vi "Load_from_Project.vi"(8 "error in (no error)":errorcluster, 9 "index":string, 10 "buildObject":T1, 11 "Class in":refnum<class "IB_DistPart.lvclass">) -> (0 "error out":errorcluster, 3 "Class out":refnum<class "IB_DistPart.lvclass">)   [LabVIEW 2020, in "IB_DistPart.lvclass"]
uses:
  <vilib>/AppBuilder/IB_Classes/DistPart/IB_DistPart.lvclass
  <vilib>/AppBuilder/IB_Classes/DistPart/IB_DistPart.lvclass/IB_DistPart.ctl
  <vilib>/AppBuilder/IB_RW_Project/IB_RW_Project_PropBag_Action.ctl
  <vilib>/AppBuilder/IB_Classes/SoftDependency/IB_SoftDependency.lvclass
  <resource>/Framework/Providers/API/ItemRef.ctl
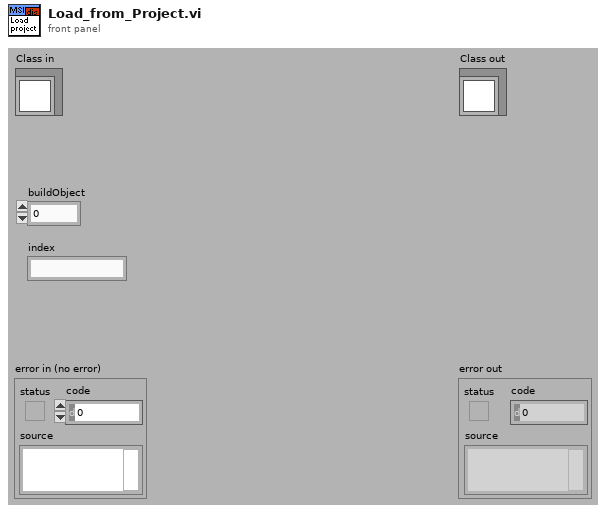
[diagram p1: front panel]
types:
  T1 = typedef "ItemRef.ctl" = u64
  T2 = typedef "IB_RW_Project_PropBag_Action.ctl" = enum16{"read", "write", "clear", "readPrevious", "writePrevious", "clearPrevious"}
  T3 = typedef "IB_RW_Project_DistPart_Data.ctl" = cluster{"ProductId":string, "FlavorId":string, "ProdName":string, "UpgradeCode":string}
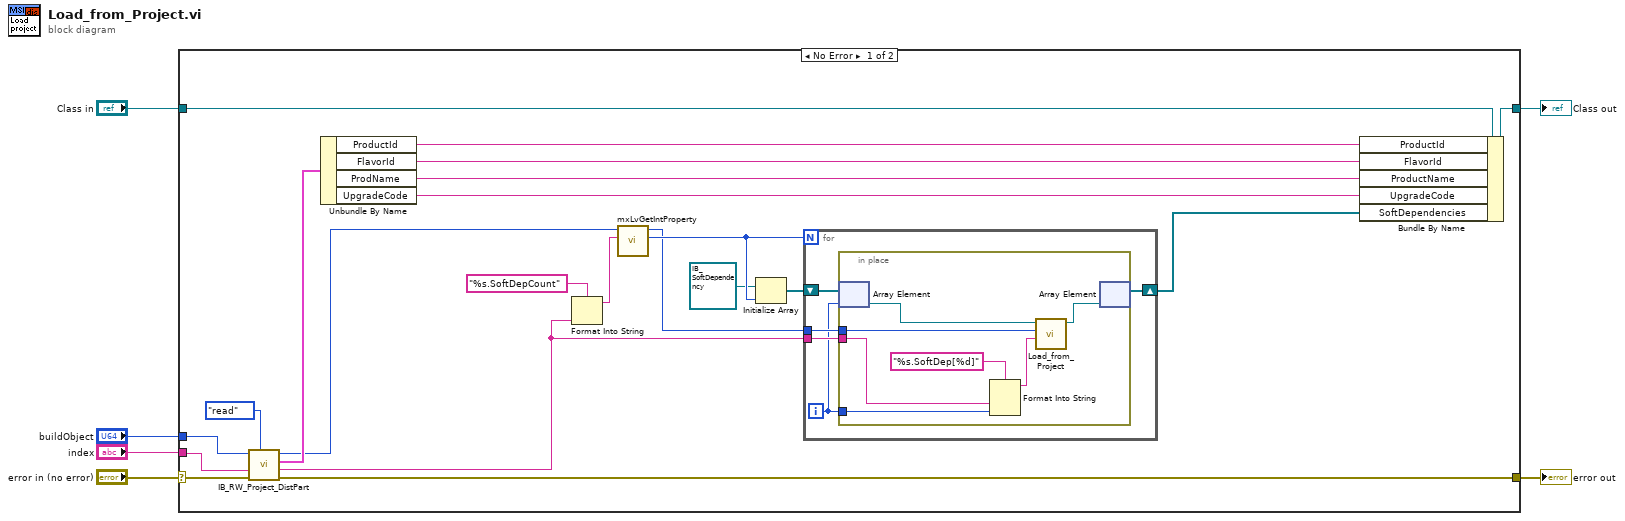
[diagram p0: block diagram]
diagram:
  n1 = case shown="No Error" "error in (no error)" {
    selector: "error in (no error)" -> [w17 w41]
    tunnel: [w16 w41] -> w5
    tunnel: [w23 w40] -> w3
    tunnel: "Class in" -> [w24 w40]
    tunnel: "buildObject" -> [w27 _]
    tunnel: "index" -> [w26 _]
    frame No Error {
      n2 = call <vilib>:"IB_RW_Project_DistPart.vi"("action"=IB_RW_Project_PropBag_Action."read", "error in (no error)"=w17, "index in"=w26, "buildObject"=w27) -> ("error out"=w16:errorcluster, "index out"=w7:string, "DistParts"=w25:T3, "buildObject out"=w9:T1)  [unwired: 1 in, 3 out]
      n3 = Unbundle By Name(w25) -> ("ProductId"=w22:string, "FlavorId"=w21:string, "ProdName"=w20:string, "UpgradeCode"=w19:string)
      n4 = Format Into String(format string="%s.SoftDepCount", w7) -> (resulting string=w11:string)  [unwired: 2 in, 1 out]
      n5 = call <resource>:"mxLvGetIntProperty.vi"("Tag"=w11, "Item"=w9) -> ("Value"=w15:i32, "Item"=w12:T1)  [unwired: 1 in, 7 out]
      n6 = Initialize Array(refnum<class "IB_SoftDependency.lvclass"> refnum ("IB_SoftDependency.lvclass"), w15) -> (w14:refnum<class "IB_SoftDependency.lvclass">[])
      n7 = for {
        N: w15 -> [_]
        tunnel: w7 -> [w32]
        tunnel: w12 -> [w31]
        shift-right: [w29] -> w8
        shift-left: w14 -> [w30]
        i -> [w28]
        n8 = in-place {
          in-place-border: w32 -> [w34]
          in-place-border: w31 -> [w39]
          in-place-border: w28 -> [w35]
          n9 = in-place-array #1(w30, w28) -> (w38:refnum<class "IB_SoftDependency.lvclass">)
          n10 = Format Into String(format string="%s.SoftDep[%d]", w34, w35) -> (resulting string=w33:string)  [unwired: 2 in, 1 out]
          n11 = call <vilib>:"Load_from_Project.vi"("index"=w33, "buildObject"=w39, "IB_SoftDependency in"=w38) -> ("IB_SoftDependency out"=w37:refnum<class "IB_SoftDependency.lvclass">)  [unwired: 1 in, 7 out]
          n12 = in-place-array #1(w37) -> (w29:refnum<class "IB_SoftDependency.lvclass">[])  [unwired: 1 out]
        }
      }
      n13 = Bundle By Name(cluster=w24, "ProductId"=w22, "FlavorId"=w21, "ProductName"=w20, "UpgradeCode"=w19, "SoftDependencies"=w8) -> (w23:refnum<class "IB_DistPart.lvclass">)
    }
    frame Error {
    }
  }
  "error out" <- w5
  "Class out" <- w3
